vi "Benchmark - Convert Pixels To Picture.vi"() -> ()   [LabVIEW 2020, in "Utility.lvlib"]
uses:
  Utility.lvlib
  e53520d9-7f1c-41dc-9216-a66112f00c7c.vi
  bd19d168-f5f9-4988-a993-845af133389d.vi
  Main/Scene/Scene.lvclass
  Benchmark/Benchmark.lvlib
  <vilib>/Analysis/NI_AALBase.lvlib
panel:
  out "Std Dev":dbl format="%.1p"
  out "Mean":dbl format="%.1p"
  out "Histogram Graph":T1(graph)
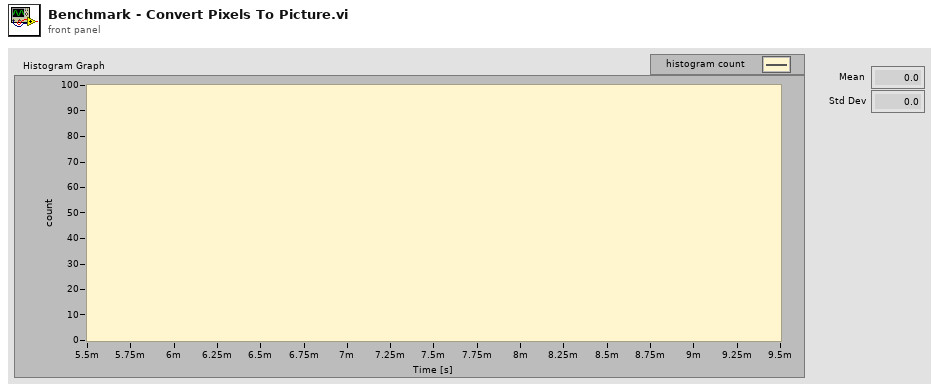
[diagram p1: front panel]
types:
  T1 = cluster{"X Values":dbl[], "Histogram: h(x)":i32[]}
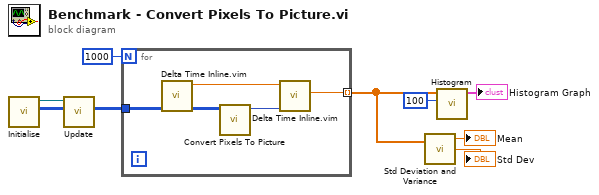
[diagram p0: block diagram]
diagram:
  n1 = call "Initialise.vi"() -> ("Pixel Data out"=w2:u32[][], "Scene out"=w3:refnum<class "Scene.lvclass">)  [unwired: 10 in]
  n2 = call "Update.vi"("Pixel Data in"=w2, "Scene in"=w3) -> ("Pixel Data out"=w1:u32[][])  [unwired: 8 in, 1 out]
  n3 = for {
    N: 1000 -> [_]
    tunnel: [w14] -> w6 mode=indexing
    tunnel: w1 -> [w12]
    n4 = call "Delta Time Inline.vim"("value in"=w12) -> ("value out"=w11:u32[][], "Relative Seconds out [s]"=w13:dbl)  [unwired: 8 in, 1 out]
    n5 = call "Convert Pixels To Picture.vi"("Pixel Data in"=w11) -> ("2D Picture"=w10:picture)  [unwired: 9 in, 1 out]
    n6 = call "Delta Time Inline.vim"("value in"=w10, "Relative Seconds in [s]"=w13) -> ("Delta Time [s]"=w14:dbl)  [unwired: 7 in, 2 out]
  }
  n7 = call <vilib>:"Std Deviation and Variance.vi"("X"=w6) -> ("mean"=→"Mean":dbl, "standard deviation"=→"Std Dev":dbl)  [unwired: 1 in, 1 out]
  n8 = call <vilib>:"Histogram.vi"("intervals"=100, "X"=w6) -> ("Histogram Graph"=→"Histogram Graph":T1)  [unwired: 6 in, 3 out]
